vi "Interpret Z Position From Raw Data.vi"   [LabVIEW 2013]
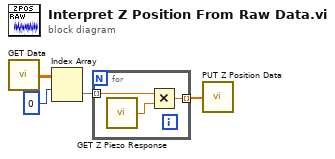
[diagram p0: block diagram]
diagram:
  n1 = call "GET Data.vi"() -> ("Data"=w1:dbl[][])
  n2 = Index Array(array=w1, index (row)=0) -> (element=w3:dbl[])  [unwired: 1 in]
  n3 = for {
    tunnel: w3 -> [w7] mode=indexing
    tunnel: [w5] -> w4 mode=indexing
    n4 = call "GET Z Piezo Response.vi"() -> ("Z Piezo Response"=w6:dbl)
    n5 = Multiply(x=w7, y=w6) -> (x*y=w5:dbl)
  }
  n6 = call "PUT Z Position Data.vi"("Z Position Data"=w4) -> ()
